vi "Sensor Demo.vi"() -> ()   [LabVIEW 2012]
uses:
  <vilib>/imath/engines/lvmath/Plug In/_Char/NIMS_CH_character datatype.ctl
  <vilib>/Utility/inputDevices.llb/closeKeyboard.vi
  <vilib>/Utility/inputDevices.llb/keyboardAcquire.vi
  <vilib>/imath/engines/lvmath/Plug In/_Char/NIMS_CH_Character RV to String.vi
  <vilib>/imath/engines/lvmath2/RunTimeEngine/NodeEndStatement/NIMS_NodeEndStatement_Output.vi
  <instcachedir>/0/NIMS_NodeEndStatement_Output_53EC0D466D134D7ABD903AC30B43404B.lvgen/NIMS_NodeEndStatement_Output_53EC0D466D134D7ABD903AC30B43404B_009.vi
  <vilib>/imath/engines/lvmath2/RunTimeEngine/ErrorHandling/NIMS_Finalize Error.vi
panel:
  in  "Data Buffer":i32=10000
  out "Live Color Reading":u32(colorbox)
  out "Identified Color":u32(colorbox)
  out "Blue?":bool
  out "Green?":bool
  out "Red?":bool
  out "Trigger?":bool
  in  "Trigger":dbl=0.3
  out "Color Sensor":T1(graph)
  out "Step 2":i64
  out "Step 1":i64
  out "Bump 2?":bool
  out "Bump 1?":bool
  out "Encoder 2":dbl
  out "Encoder 1":dbl
  out "Bump 2":dbl
  out "Bump 1":dbl
  out "Battery":dbl(slide) scale=0.0..10.0
  out "Analog Encoder [Sonar Eventually]":dbl[](graph)
  out "IR 1":dbl[](graph)
  out "Lidar 2":dbl[](graph)
  out "Lidar 1":dbl[](graph)
  out "RECEIVING SONAR":bool
  out "RECEIVING BUMP 2":bool
  out "RECEIVING BATTERY":bool
  out "RCV'G COLOR BLUE":bool
  out "RCV'G COLOR GREEN":bool
  out "RCV'G COLOR RED":bool
  out "RECEIVING BUMP 1":bool
  out "RCV'G ENCODER 2":bool
  out "RCV'G ENCODER 1":bool
  out "RECEIVING IR 1":bool
  out "RECEIVING LIDAR 2":bool
  in  "MANUAL \nOVERRIDE":bool=TRUE
  out "Right Speed":i32(knob) scale=1000.0..2000.0
  out "Left Speed":i32(knob) scale=1000.0..2000.0
  in  "Servo 1":i32(slide)=1500 scale=500.0..2500.0
  in  "Step Size":i32=5
  out "Speed                    Balance":i32(knob) scale=-1000.0..1000.0
  in  "Servo 2":i32(slide)=1500 scale=500.0..2500.0
  out "Servo One":i32
  out "Servo Two":i32
  out "Left Motor":i32
  out "Right Motor":i32
  in  "PC Status":i32=1
  out "XBEE Working":bool
  out "return count":u32
  out "Sent from XBEE":string
  out "bytes written":u32
  in  "Send to XBEE":string
  in  "VISA resource name":refnum<visa-resource-name>="COM10"
  in  "FULL STOP":bool
  in  "ESTOP":bool
  out "RECEIVING LIDAR 1":bool
  # "Digital Sensors"
  # "Color\nProcessing"
  # "Red"
  # "Green"
  # "Blue"
  # "Sends stop code to \nXBEE. Assumes on-\nRobot code will stop."
  # "Ends all looped\nprocesses."
  # "A0"
  # "D2"
  # "A7"
  # "A1"
  # "D3"
  # "A6"
  # "A5"
  # "A2"
  # "D4"
  # "A4"
  # "A3"
  # "D5"
  # "MANUAL ACTUATION CONTROLS"
  # "Affects weight of \na single key input."
  # "Controls:\nUse W/S to independently\ncontrol port speed.\nUse I/K to independently\ncontrol starboard speed.\nUse arrow keys to jointly\ncontrol motor speeds.\n\nUSE ESCAPE TO KILL MOTORS."
  # "ACTUAL PWM WIDTHS SENT"
  # "XBEE COMMUNICATION"
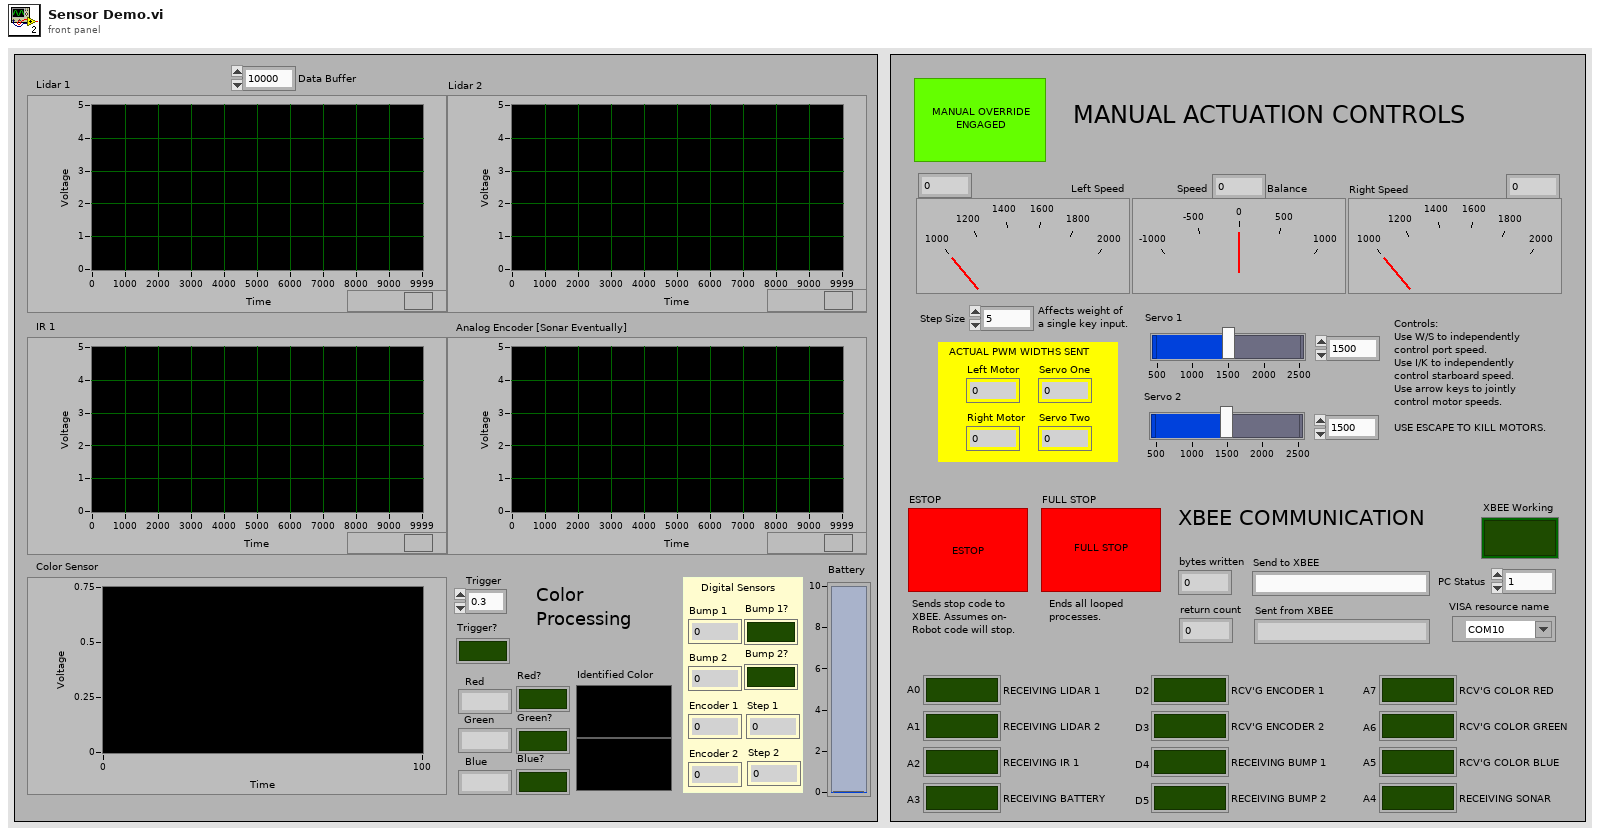
[diagram p1: front panel]
types:
  T1 = cluster{"Voltage":dbl, "Voltage":dbl, "Voltage":dbl}
  T2 = enum16{"0", "1", "2", "3", "4", "5", "6", "7", "8", "9", "A", "B", "C", "D", "E", "F", "G", "H", "I", "J", "K", "L", "M", "N", "O", "P", "Q", "R", "S", "T", "U", "V", "W", "X", "Y", "Z", "F1", "F2", "F3", "F4", "F5", "F6", "F7", "F8", "F9", "F10", "F11", "F12", "F13", "F14", "F15", "ADD", "BACK", "BACKSLASH", "CAPITAL", "COMMA", "DECIMAL", "DELETE", "DIVIDE", "DOWN", "END", "EQUALS", "ESCAPE", "GRAVE (`)", "HOME", "INSERT", "LBRACKET", "LCONTROL", "LEFT", "L ALT", "LSHIFT", "LWIN", "MINUS", "MULTIPLY", "NEXT", "NUMLOCK", "NUMPAD_0", "NUMPAD_1", "NUMPAD_2", "NUMPAD_3", "NUMPAD_4", "NUMPAD_5", "NUMPAD_6", "NUMPAD_7", "NUMPAD_8", "NUMPAD_9", "PAUSE", "PERIOD", "PRIOR (PG UP)", "RBRACKET", "RCONTROL", "RETURN", "RIGHT", "R ALT", "RSHIFT", "RWIN", "SCROLL", "SEMICOLON", "SLASH", "SPACE", "SUBTRACT", "TAB", "UP", "ENTER (num pad)", "' (quote)"}[]
  T3 = enum16{"0", "1", "2", "3", "4", "5", "6", "7", "8", "9", "A", "B", "C", "D", "E", "F", "G", "H", "I", "J", "K", "L", "M", "N", "O", "P", "Q", "R", "S", "T", "U", "V", "W", "X", "Y", "Z", "F1", "F2", "F3", "F4", "F5", "F6", "F7", "F8", "F9", "F10", "F11", "F12", "F13", "F14", "F15", "ADD", "BACK", "BACKSLASH", "CAPITAL", "COMMA", "DECIMAL", "DELETE", "DIVIDE", "DOWN", "END", "EQUALS", "ESCAPE", "GRAVE (`)", "HOME", "INSERT", "LBRACKET", "LCONTROL", "LEFT", "L ALT", "LSHIFT", "LWIN", "MINUS", "MULTIPLY", "NEXT", "NUMLOCK", "NUMPAD_0", "NUMPAD_1", "NUMPAD_2", "NUMPAD_3", "NUMPAD_4", "NUMPAD_5", "NUMPAD_6", "NUMPAD_7", "NUMPAD_8", "NUMPAD_9", "PAUSE", "PERIOD", "PRIOR (PG UP)", "RBRACKET", "RCONTROL", "RETURN", "RIGHT", "R ALT", "RSHIFT", "RWIN", "SCROLL", "SEMICOLON", "SLASH", "SPACE", "SUBTRACT", "TAB", "UP", "ENTER (num pad)", "' (quote)"}
  T4 = typedef "NIMS_CH_character datatype.ctl" = cluster{"Numeric":u8}
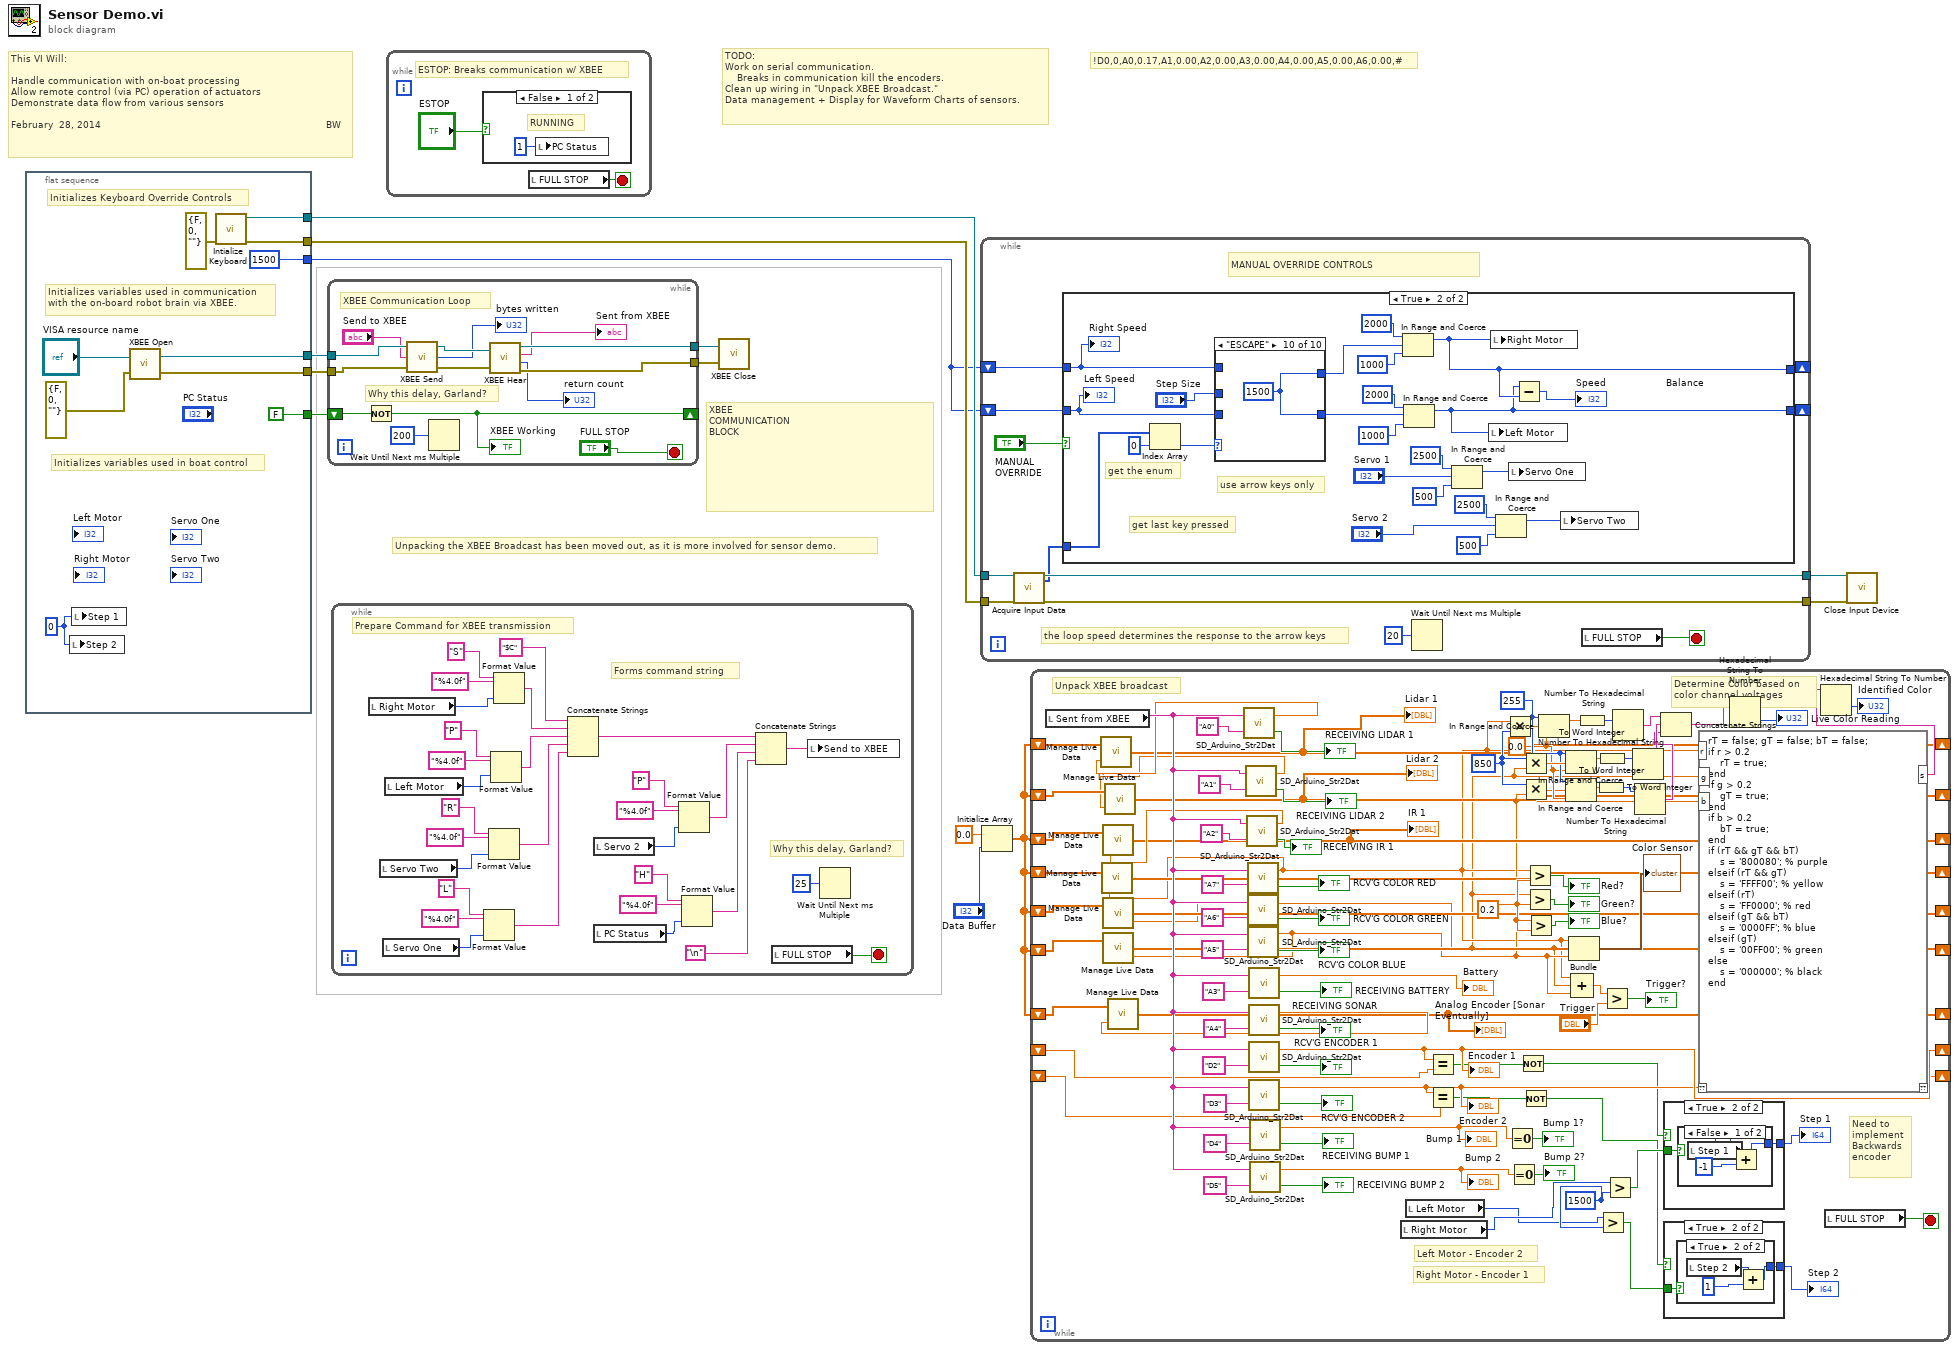
[diagram p0: block diagram]
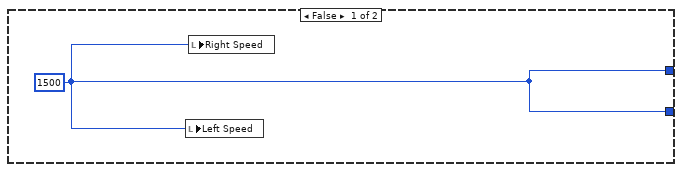
[diagram p2: hidden frame]
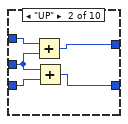
[diagram p4: hidden frame]
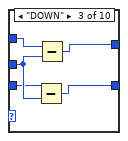
[diagram p5: hidden frame]
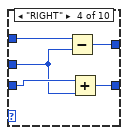
[diagram p6: hidden frame]
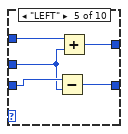
[diagram p7: hidden frame]
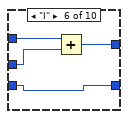
[diagram p8: hidden frame]
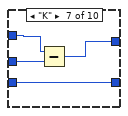
[diagram p9: hidden frame]
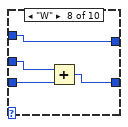
[diagram p10: hidden frame]
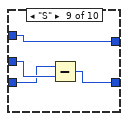
[diagram p11: hidden frame]
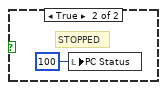
[diagram p12: hidden frame]
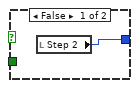
[diagram p13: hidden frame]
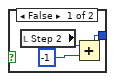
[diagram p14: hidden frame]
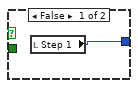
[diagram p15: hidden frame]
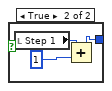
[diagram p16: hidden frame]
diagram:
  # "TODO: \nWork on serial communication.\n    Breaks in communication kill the encoders.\nClean up wiring in \"Unpack XBEE Broadcast.\"\nData management + Display for Waveform Charts of sensors."
  # "Unpacking the XBEE Broadcast has been moved out, as it is more involved for sensor demo."
  # "!D0,0,A0,0.17,A1,0.00,A2,0.00,A3,0.00,A4,0.00,A5,0.00,A6,0.00,#"
  # "XBEE \nCOMMUNICATION\nBLOCK"
  # "This VI Will:\n\nHandle communication with on-boat processing\nAllow remote control (via PC) operation of actuators\nDemonstrate data flow from various sensors\n\nFebruary  28, 2014                                                                           BW"
  n1 = flat-sequence {
    tunnel: [w21] -> w13
    tunnel: [w20] -> w12
    tunnel: [FALSE] -> w9
    tunnel: [w17] -> w6
    tunnel: [w16] -> w5
    tunnel: [1500] -> w4
    frame #0 {
      w14 = 0
      # "Initializes Keyboard Override Controls"
      # "Initializes variables used in boat control"
      # "Initializes variables used in communication\nwith the on-board robot brain via XBEE."
      n2 = local write "Step 2"(w14) -> ()
      n3 = local write "Step 1"(w14) -> ()
      n4 = call "XBEE Open.vi"("error in"=errorcluster {"status"=FALSE, "code"=0, "source"=""}, "VISA resource name"="VISA resource name") -> ("error out"=w20:errorcluster, "VISA resource name out"=w21:refnum<visa-resource-name>)
      n5 = call <vilib>:"Intialize Keyboard.vi"("error in (no error)"=errorcluster {"status"=FALSE, "code"=0, "source"=""}) -> ("error out"=w16:errorcluster, "device ID"=w17:refnum<k1>)  [unwired: 9 in]
    }
  }
  n6 = while {
    tunnel: w13 -> [w37]
    tunnel: w12 -> [w36]
    tunnel: [w31] -> w11
    tunnel: [w30] -> w10
    shift-right: [w25] -> _
    shift-left: w9 -> [w27]
    stop <- "FULL STOP" stop-if-true
    # "Why this delay, Garland?"
    # "XBEE Communication Loop"
    n7 = Not(x=w27) -> (.not. x?=w25:bool)
    "XBEE Working" <- w25
    n8 = call "XBEE Send.vi"("error in (no error)"=w36, "String"="Send to XBEE", "VISA resource name"=w37) -> ("error out"=w33:errorcluster, "return count"=→"bytes written":u32, "VISA resource name out"=w34:refnum<visa-resource-name>)
    n9 = Wait Until Next ms Multiple(millisecond multiple=200) -> ()  [unwired: 1 out]
    n10 = call "XBEE Hear.vi"("VISA resource name"=w34, "error in (no error)"=w33) -> ("VISA resource name out"=w31:refnum<visa-resource-name>, "String Received"=→"Sent from XBEE":string, "return count"=→"return count":u32, "error out"=w30:errorcluster)
  }
  n11 = while {
    stop <- w67 stop-if-true
    # "Why this delay, Garland?"
    # "Prepare Command for XBEE transmission"
    # "Forms command string"
    n12 = local read "Right Motor"() -> (w64:i32)
    n13 = local read "Servo Two"() -> (w55:i32)
    n14 = local read "Servo One"() -> (w52:i32)
    n15 = local read "Left Motor"() -> (w61:i32)
    n16 = Format Value(string ("")="L", format string="%4.0f", value (0)=w52) -> (output string=w50:string)
    n17 = Format Value(string ("")="R", format string="%4.0f", value (0)=w55) -> (output string=w51:string)
    n18 = Format Value(string ("")="P", format string="%4.0f", value (0)=w61) -> (output string=w58:string)
    n19 = Format Value(string ("")="S", format string="%4.0f", value (0)=w64) -> (output string=w59:string)
    n20 = Concatenate Strings("$C", w59, w58, w51, w50) -> (w42:string)
    n21 = local read "Servo 2"() -> (w46:i32)
    n22 = local read "PC Status"() -> (w43:i32)
    n23 = Format Value(string ("")="P", format string="%4.0f", value (0)=w46) -> (output string=w41:string)
    n24 = Format Value(string ("")="H", format string="%4.0f", value (0)=w43) -> (output string=w40:string)
    n25 = Concatenate Strings(w42, w41, w40, "\n") -> (w47:string)
    n26 = local read "FULL STOP"() -> (w67:bool)
    n27 = local write "Send to XBEE"(w47) -> ()
    n28 = Wait Until Next ms Multiple(millisecond multiple=u32 25) -> ()  [unwired: 1 out]
  }
  n29 = while {
    stop <- w69 stop-if-true
    # "ESTOP: Breaks communication w/ XBEE"
    n30 = case shown="False" "ESTOP" {
      frame False {
        # "RUNNING"
        n31 = local write "PC Status"(1 ("PC Status")) -> ()
      }
      frame True {
        # "STOPPED"
        n32 = local write "PC Status"(100) -> ()
      }
    }
    n33 = local read "FULL STOP"() -> (w69:bool)
  }
  n34 = call "XBEE Close.vi"("error in (no error)"=w10, "VISA resource name"=w11) -> ()
  n35 = while {
    tunnel: [w83] -> w7
    tunnel: [w82] -> w8
    shift-right: [w76] -> _
    shift-left: w4 -> [w79]
    shift-right: [w75] -> _
    shift-left: w4 -> [w78]
    tunnel: w6 -> [w74]
    tunnel: w5 -> [w73]
    stop <- w77 stop-if-true
    # "MANUAL OVERRIDE CONTROLS"
    # "the loop speed determines the response to the arrow keys"
    n36 = call-poly <vilib>:"Acquire Input Data.vi"("device ID"=w74, "error in (no error)"=w73) -> ("device ID"=w82:refnum<k1>, "keys pressed"=w81:T2, "error out"=w83:errorcluster)  [unwired: 15 in]
    n37 = case shown="True" "MANUAL \nOVERRIDE" {
      tunnel: w81 -> [_ w107]
      tunnel: w79 -> [_ w104]
      tunnel: w78 -> [_ w103]
      tunnel: [w84 w91] -> w76
      tunnel: [w84 w90] -> w75
      frame False {
        w84 = 1500
        n38 = local write "Left Speed"(w84) -> ()
        n39 = local write "Right Speed"(w84) -> ()
      }
      frame True {
        # "use arrow keys only"
        # "get the enum"
        # "get last key pressed"
        n40 = Index Array(array=w107, index=0) -> (element=w105:T3)
        n41 = case shown="\"ESCAPE\"" w105 {
          tunnel: w104 -> [w109 w114 w119 w121 w126 w133 w135 w138 w142 _]
          tunnel: [w109 w113 w118 w122 w127 w132 w134 w138 w142 w146] -> w102
          tunnel: w103 -> [w108 w111 w116 w124 w128 w130 w137 w140 w144 _]
          tunnel: [w108 w110 w115 w123 w129 w130 w137 w139 w143 w146] -> w93
          tunnel: "Step Size" -> [_ w112 w117 w120 w125 w131 w136 w141 w145 _]
          frame "0", Default {
          }
          frame "UP" {
            n42 = Add(x=w114, y=w112) -> (x+y=w113:i32)
            n43 = Add(x=w112, y=w111) -> (x+y=w110:i32)
          }
          frame "DOWN" {
            n44 = Subtract(x=w116, y=w117) -> (x-y=w115:i32)
            n45 = Subtract(x=w119, y=w117) -> (x-y=w118:i32)
          }
          frame "RIGHT" {
            n46 = Subtract(x=w121, y=w120) -> (x-y=w122:i32)
            n47 = Add(x=w124, y=w120) -> (x+y=w123:i32)
          }
          frame "LEFT" {
            n48 = Subtract(x=w128, y=w125) -> (x-y=w129:i32)
            n49 = Add(x=w126, y=w125) -> (x+y=w127:i32)
          }
          frame "I" {
            n50 = Add(x=w133, y=w131) -> (x+y=w132:i32)
          }
          frame "K" {
            n51 = Subtract(x=w135, y=w136) -> (x-y=w134:i32)
          }
          frame "W" {
            n52 = Add(x=w141, y=w140) -> (x+y=w139:i32)
          }
          frame "S" {
            n53 = Subtract(x=w144, y=w145) -> (x-y=w143:i32)
          }
          frame "ESCAPE" {
            w146 = 1500
          }
        }
        n54 = In Range and Coerce(upper limit=2000, x=w102, lower limit=1000) -> (coerced(x)=w91:i32)  [unwired: 1 out]
        n55 = In Range and Coerce(upper limit=2000, x=w93, lower limit=1000) -> (coerced(x)=w90:i32)  [unwired: 1 out]
        n56 = In Range and Coerce(upper limit=2500, x="Servo 1", lower limit=500) -> (coerced(x)=w89:i32)  [unwired: 1 out]
        n57 = local write "Left Motor"(w90) -> ()
        n58 = local write "Right Motor"(w91) -> ()
        n59 = In Range and Coerce(upper limit=2500, x="Servo 2", lower limit=500) -> (coerced(x)=w86:i32)  [unwired: 1 out]
        n60 = local write "Servo One"(w89) -> ()
        n61 = Subtract(x=w90, y=w91) -> (x-y=→"Speed                    Balance":i32)
        n62 = local write "Servo Two"(w86) -> ()
        "Right Speed" <- w104
        "Left Speed" <- w103
      }
    }
    n63 = Wait Until Next ms Multiple(millisecond multiple=u32 20) -> ()  [unwired: 1 out]
    n64 = local read "FULL STOP"() -> (w77:bool)
  }
  n65 = Initialize Array(0.0 ("element"), "Data Buffer") -> (w1:dbl[])
  n66 = while {
    shift-right: [w180] -> _
    shift-left: _ -> [w181]
    shift-right: [w179] -> _
    shift-left: _ -> [w182]
    shift-right: [w174] -> _
    shift-left: w1 -> [w176]
    shift-right: [w163] -> _
    shift-left: w1 -> [w173]
    shift-right: [w161] -> _
    shift-left: w1 -> [w169]
    shift-right: [w167] -> _
    shift-left: w1 -> [w170]
    shift-right: [w166] -> _
    shift-left: w1 -> [w171]
    shift-right: [w165] -> _
    shift-left: w1 -> [w172]
    shift-right: [w159] -> _
    shift-left: w1 -> [w168]
    stop <- w240 stop-if-true
    w156 = 1500
    w195 = 0.0 ("lower limit")
    w196 = 255
    w199 = 850
    w206 = 0.2
    # "Right Motor - Encoder 1"
    # "Left Motor - Encoder 2"
    # "Need to\nimplement\nBackwards\nencoder"
    # "Determine Color based on \ncolor channel voltages"
    # "Unpack XBEE broadcast"
    n67 = local read "Sent from XBEE"() -> (w216:string)
    n68 = call "SD_Arduino_Str2Dat.vi"("Arbotix Pin"="A0", "String from Robot"=w216) -> ("Pin Valid?"=→"RECEIVING LIDAR 1":bool, "Voltage"=w175:dbl)
    n69 = call "Manage Live Data.vi"("New Data Point"=w175, "Array"=w176) -> ("Updated Array"=w174:dbl[])
    "Lidar 1" <- w174
    n70 = call "SD_Arduino_Str2Dat.vi"("Arbotix Pin"="A1", "String from Robot"=w216) -> ("Pin Valid?"=→"RECEIVING LIDAR 2":bool, "Voltage"=w164:dbl)
    n71 = call "Manage Live Data.vi"("New Data Point"=w164, "Array"=w173) -> ("Updated Array"=w163:dbl[])
    "Lidar 2" <- w163
    n72 = call "SD_Arduino_Str2Dat.vi"("Arbotix Pin"="A2", "String from Robot"=w216) -> ("Pin Valid?"=→"RECEIVING IR 1":bool, "Voltage"=w162:dbl)
    n73 = call "Manage Live Data.vi"("New Data Point"=w162, "Array"=w169) -> ("Updated Array"=w161:dbl[])
    "IR 1" <- w161
    n74 = call "SD_Arduino_Str2Dat.vi"("Arbotix Pin"="A7", "String from Robot"=w216) -> ("Pin Valid?"=→"RCV'G COLOR RED":bool, "Voltage"=w155:dbl)
    n75 = call "Manage Live Data.vi"("New Data Point"=w155, "Array"=w170) -> ("Updated Array"=w167:dbl[])
    n76 = call "SD_Arduino_Str2Dat.vi"("Arbotix Pin"="A6", "String from Robot"=w216) -> ("Pin Valid?"=→"RCV'G COLOR GREEN":bool, "Voltage"=w154:dbl)
    n77 = call "Manage Live Data.vi"("New Data Point"=w154, "Array"=w171) -> ("Updated Array"=w166:dbl[])
    n78 = call "SD_Arduino_Str2Dat.vi"("Arbotix Pin"="A5", "String from Robot"=w216) -> ("Pin Valid?"=→"RCV'G COLOR BLUE":bool, "Voltage"=w158:dbl)
    n79 = call "Manage Live Data.vi"("New Data Point"=w158, "Array"=w172) -> ("Updated Array"=w165:dbl[])
    n80 = call "SD_Arduino_Str2Dat.vi"("Arbotix Pin"="A3", "String from Robot"=w216) -> ("Pin Valid?"=→"RECEIVING BATTERY":bool, "Voltage"=→"Battery":dbl)
    n81 = call "SD_Arduino_Str2Dat.vi"("Arbotix Pin"="A4", "String from Robot"=w216) -> ("Pin Valid?"=→"RECEIVING SONAR":bool, "Voltage"=w160:dbl)
    n82 = call "Manage Live Data.vi"("New Data Point"=w160, "Array"=w168) -> ("Updated Array"=w159:dbl[])
    "Analog Encoder [Sonar Eventually]" <- w159
    n83 = call "SD_Arduino_Str2Dat.vi"("Arbotix Pin"="D2", "String from Robot"=w216) -> ("Pin Valid?"=→"RCV'G ENCODER 1":bool, "Voltage"=w180:dbl)
    "Encoder 1" <- w180
    n84 = call "SD_Arduino_Str2Dat.vi"("Arbotix Pin"="D3", "String from Robot"=w216) -> ("Pin Valid?"=→"RCV'G ENCODER 2":bool, "Voltage"=w179:dbl)
    "Encoder 2" <- w179
    n85 = call "SD_Arduino_Str2Dat.vi"("Arbotix Pin"="D4", "String from Robot"=w216) -> ("Pin Valid?"=→"RECEIVING BUMP 1":bool, "Voltage"=w201:dbl)
    "Bump 1" <- w201
    n86 = call "SD_Arduino_Str2Dat.vi"("Arbotix Pin"="D5", "String from Robot"=w216) -> ("Pin Valid?"=→"RECEIVING BUMP 2":bool, "Voltage"=w200:dbl)
    "Bump 2" <- w200
    n87 = local read "Right Motor"() -> (w148:i32)
    n88 = local read "Left Motor"() -> (w147:i32)
    n89 = Equal?(x=w180, y=w181) -> (x = y?=w178:bool)
    n90 = Equal?(x=w179, y=w182) -> (x = y?=w177:bool)
    n91 = Multiply(x=w155, y=w199) -> (x*y=w198:dbl)
    n92 = Equal To 0?(x=w201) -> (x = 0?=→"Bump 1?":bool)
    n93 = Equal To 0?(x=w200) -> (x = 0?=→"Bump 2?":bool)
    n94 = Not(x=w178) -> (.not. x?=w152:bool)
    n95 = Multiply(x=w199, y=w154) -> (x*y=w197:dbl)
    n96 = Multiply(x=w199, y=w158) -> (x*y=w194:dbl)
    n97 = Not(x=w177) -> (.not. x?=w150:bool)
    n98 = Greater?(x=w155, y=w206) -> (0:→"Red?":bool)
    n99 = Greater?(x=w154, y=w206) -> (0:→"Green?":bool)
    n100 = Greater?(x=w158, y=w206) -> (0:→"Blue?":bool)
    n101 = In Range and Coerce(upper limit=w196, x=w198, lower limit=w195) -> (coerced(x)=w193:dbl)  [unwired: 1 out]
    n102 = In Range and Coerce(upper limit=w196, x=w197, lower limit=w195) -> (coerced(x)=w192:dbl)  [unwired: 1 out]
    n103 = In Range and Coerce(upper limit=w196, x=w194, lower limit=w195) -> (coerced(x)=w191:dbl)  [unwired: 1 out]
    n104 = Bundle("Voltage"=w155, "Voltage"=w154, "Voltage"=w158) -> (→"Color Sensor":T1)  [unwired: 1 in]
    n105 = Compound Arithmetic op=ADD(w155, w154, w158) -> (w212:dbl)
    n106 = To Word Integer(number=w193) -> (16bit integer=w188:i16)
    n107 = To Word Integer(number=w191) -> (16bit integer=w190:i16)
    n108 = To Word Integer(number=w192) -> (16bit integer=w189:i16)
    n109 = Greater?(x=w147, y=w156) -> (0:w151:bool)
    n110 = Greater?(x=w212, y="Trigger") -> (0:→"Trigger?":bool)
    n111 = Greater?(x=w148, y=w156) -> (0:w153:bool)
    n112 = Number To Hexadecimal String(2:w188) -> (0:w187:string)  [unwired: 1 in]
    n113 = Number To Hexadecimal String(2:w189) -> (0:w186:string)  [unwired: 1 in]
    n114 = Number To Hexadecimal String(2:w190) -> (0:w185:string)  [unwired: 1 in]
    n115 = Concatenate Strings(w187, w186, w185) -> (w184:string)
    n116 = case shown="True" w152 {
      tunnel: [w250 w252] -> w157
      tunnel: w153 -> [_ w251]
      frame False {
        n117 = local read "Step 1"() -> (w250:i64)
      }
      frame True {
        n118 = case shown="False" w251 {
          tunnel: [w254 w256] -> w252
          frame False {
            n119 = local read "Step 1"() -> (w253:i64)
            n120 = Add(x=w253, y=-1) -> (x+y=w254:i64)
          }
          frame True {
            n121 = local read "Step 1"() -> (w258:i64)
            n122 = Add(x=w258, y=1) -> (x+y=w256:i64)
          }
        }
      }
    }
    "Step 1" <- w157
    n123 = case shown="True" w150 {
      tunnel: w151 -> [_ w243]
      tunnel: [w241 w242] -> w149
      frame False {
        n124 = local read "Step 2"() -> (w241:i64)
      }
      frame True {
        n125 = case shown="True" w243 {
          tunnel: [w244 w247] -> w242
          frame False {
            n126 = local read "Step 2"() -> (w245:i64)
            n127 = Add(x=w245, y=-1) -> (x+y=w244:i64)
          }
          frame True {
            n128 = local read "Step 2"() -> (w249:i64)
            n129 = Add(x=w249, y=1) -> (x+y=w247:i64)
          }
        }
      }
    }
    "Step 2" <- w149
    n130 = mathscript code="rT = false; gT = false; bT = false;\nif r > 0.2\n    rT = true; \nend\nif g > 0.2\n    gT = true;\nend\nif b > 0.2\n    bT = true;\nend\nif (rT && gT && bT)\n    s = '800080'; % purple\nelseif (rT && gT)\n    s = 'FFFF00'; % yellow\nelseif (rT)\n    s = 'FF0000'; % red\nelseif (gT && bT)\n    s = '0000FF'; % blue\nelseif (gT)\n    s = '00FF00'; % green\nelse\n    s = '000000'; % black\nend"("r"=w155, "g"=w154, "b"=w158) -> ("s"=w204:string)  [unwired: 1 in, 1 out]
    n131 = Hexadecimal String To Number(string=w184) -> (number=→"Live Color Reading":u32)  [unwired: 2 in, 1 out]
    n132 = Hexadecimal String To Number(string=w204) -> (number=→"Identified Color":u32)  [unwired: 2 in, 1 out]
    n133 = local read "FULL STOP"() -> (w240:bool)
  }
  n134 = call-poly <vilib>:"Close Input Device.vi"("error in (no error)"=w7, "device ID"=w8) -> ()  [unwired: 8 in, 1 out]
